vi "Object_Track_Webcam_RIO.vi"() -> ()   [LabVIEW 2017]
doc: "This example demonstrates the Traditional MeanShift algorithm to track an object in the image."
uses:
  <vilib>/NI_Real-Time Target Support.lvlib
panel:
  out "CPU Load":dbl(graph)
  in  "AVI File Path":path=path "/home/lvuser/Traffic.avi"
  in  "Stop":bool
  in  "Delay (s.)":dbl(slide)=0.2040816326530612 scale=0.0..2.0
  out "Image":T1(plugin-control)
  # "Overview: Demonstrate the Traditional MeanShift algorithm to track an object in the image.\nRequirements: LabVIEW Full Development System and Vision Development Module.\nInstructions: Run the VI."
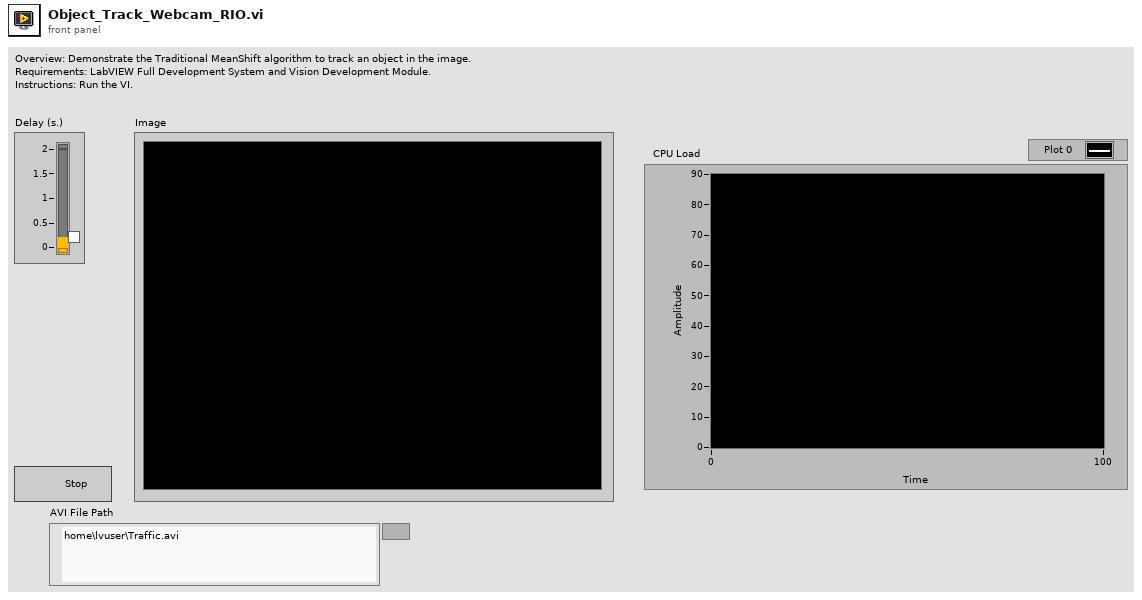
[diagram p1: front panel]
types:
  T1 = typedef "IMAQ Image.ctl" = refnum<image>
  T2 = cluster{"Number of Histogram Bins":i32, "Blending Parameter (%)":dbl, "Maximum Iterations":i32}
  T3 = typedef "IMAQ Object Tracking Session.ctl" = refnum<k20>
  T4 = typedef "IMAQ AVI2 Refnum.ctl" = refnum<k20>
  T5 = typedef "Image Type" = u32
  T6 = typedef "IMAQ Rectangle" = cluster{"Left":i32, "Top":i32, "Right":i32, "Bottom":i32, "Rotation":dbl}
  T7 = typedef "ROI Descriptor" = cluster{"Global Rectangle":i32[], "Contours":cluster{"ID":enum32{"External", "Internal"}, "Type":u32, "Coordinates":i32[]}[]}
  T8 = cluster{"Label":string, "Score":i32, "Angle":dbl, "Location":cluster{"X":dbl, "Y":dbl}, "Bounding Box":cluster{"X":dbl, "Y":dbl}[], "Object Found?":bool}[]
  T9 = cluster{"Label":string, "Score":i32, "Angle":dbl, "Location":cluster{"X":dbl, "Y":dbl}, "Bounding Box":cluster{"X":dbl, "Y":dbl}[], "Object Found?":bool}
  T10 = typedef "NI_Real-Time Target Support.lvlib/RT CPU Load.ctl" = cluster{"Total (%)":dbl, "Time Critical (%)":dbl, "Timed Structures (%)":dbl, "High (%)":dbl, "Above Normal (%)":dbl, "Normal (%)":dbl, "Background (%)":dbl, "Idle (%)":dbl, "ISR (%)":dbl}
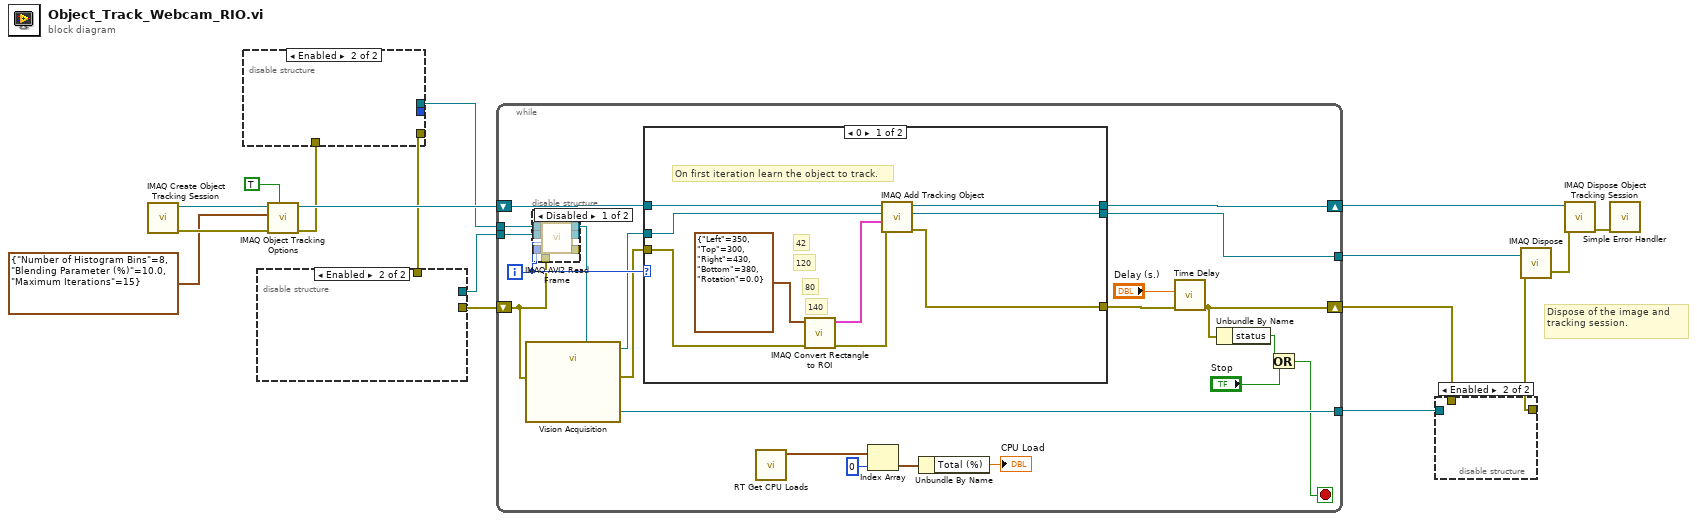
[diagram p0: block diagram]
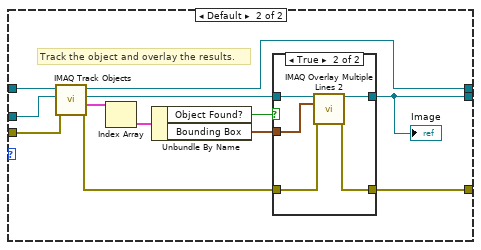
[diagram p3: hidden frame]
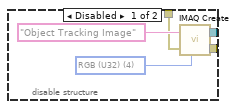
[diagram p5: hidden frame]
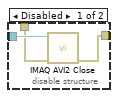
[diagram p6: hidden frame]
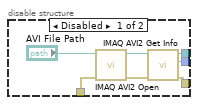
[diagram p7: hidden frame]
diagram:
  # "Dispose of the image and tracking session."
  n1 = call "IMAQ Create Object Tracking Session"() -> ("error out"=w10:errorcluster, "Object Tracking Session"=w13:T3)  [unwired: 1 in, 9 out]
  n2 = call-poly "IMAQ Object Tracking Options"("Get/Set (Get)"=TRUE, "error in (no error)"=w10, "Mean Shift Options in"=T2 {"Number of Histogram Bins"=8, "Blending Parameter (%)"=10.0, "Maximum Iterations"=15}, "Object Tracking Session In"=w13) -> ("error out"=w9:errorcluster, "Object Tracking Session Out"=w12:T3)  [unwired: 5 in, 1 out]
  n3 = disable-structure shown="Enabled" {
    disable-tunnel: w9 -> [w24 _]
    disable-tunnel: [w21 _] -> _
    disable-tunnel: [w20 _] -> w8
    disable-tunnel: [w19 _] -> w7
    frame Disabled {
      n4 = call "IMAQ AVI2 Open"("error in (no error)"=w24, "AVI File Path"="AVI File Path") -> ("error out"=w22:errorcluster, "AVI Refnum"=w23:T4)  [unwired: 8 in]
      n5 = call "IMAQ AVI2 Get Info"("error in (no error)"=w22, "AVI Refnum"=w23) -> ("error out"=w20:errorcluster, "Number of Frames"=w21:u32, "AVI Refnum (duplicate)"=w19:T4)  [unwired: 5 in, 2 out]
    }
    frame Enabled {
    }
  }
  n6 = disable-structure shown="Enabled" {
    disable-tunnel: w8 -> [w28 _]
    disable-tunnel: [w26 _] -> w6
    disable-tunnel: [w25 _] -> w5
    frame Disabled {
      w27 = T5 4 items=["Grayscale (U8)", "Grayscale (I16)", "Grayscale (SGL)", "Complex (CSG)", "RGB (U32)", "HSL (U32)", "RGB (U64)", "Grayscale (U16)"] ("Image Type")
      n7 = call "IMAQ Create"("Image Name"="Object Tracking Image", "Image Type"=w27, "error in (no error)"=w28) -> ("New Image"=w26:T1, "error out"=w25:errorcluster)  [unwired: 2 in]
    }
    frame Enabled {
    }
  }
  n8 = while {
    tunnel: [w48] -> w17
    shift-right: [w46] -> w16
    shift-left: w12 -> [w47]
    tunnel: w7 -> [w44]
    tunnel: w6 -> [w43]
    shift-right: [w32] -> w3
    shift-left: w5 -> [w35]
    tunnel: [w40] -> w4
    i -> [w42]
    stop <- w31 stop-if-true
    n9 = call "Vision Acquisition"("error in"=w35) -> ("Image Out"=w34:T1, "error out"=w33:errorcluster)  [unwired: 24 in, 1 out]
    n10 = disable-structure shown="Disabled" {
      disable-tunnel: w44 -> [w56 _]
      disable-tunnel: w43 -> [w55 _]
      disable-tunnel: [w54 _] -> _
      disable-tunnel: [w53 _] -> _
      disable-tunnel: w42 -> [w52 _]
      disable-tunnel: w35 -> [w51 _]
      disable-tunnel: [w50 _] -> w40
      frame Disabled {
        n11 = call "IMAQ AVI2 Read Frame"("error in (no error)"=w51, "Frame Number"=w52, "Image"=w55, "AVI Refnum"=w56) -> ("error out"=w53:errorcluster, "Image Out"=w54:T1, "AVI Refnum (duplicate)"=w50:T4)  [unwired: 5 in]
      }
      frame Enabled {
      }
    }
    n12 = case shown="0" w42 {
      tunnel: [w62 w77] -> w46
      tunnel: [w64 w74] -> w48
      tunnel: [w63 w70] -> w30
      tunnel: w47 -> [w65 w72]
      tunnel: w34 -> [w61 w68]
      tunnel: w33 -> [w60 w67]
      frame 0 {
        # "140"
        # "80"
        # "42"
        # "120"
        # "On first iteration learn the object to track."
        n13 = call "IMAQ Convert Rectangle to ROI"("error in (no error)"=w60, "Rectangle"=T6 {"Left"=350, "Top"=300, "Right"=430, "Bottom"=380, "Rotation"=0.0}) -> ("error out"=w59:errorcluster, "ROI Descriptor"=w58:T7)  [unwired: 7 in]
        n14 = call "IMAQ Add Tracking Object"("error in (no error)"=w59, "ROI Descriptor"=w58, "Image"=w61, "Object Tracking Session In"=w65) -> ("error out"=w63:errorcluster, "Image (duplicate)"=w64:T1, "Object Tracking Session Out"=w62:T3)  [unwired: 1 in, 4 out]
      }
      frame Default {
        # "Track the object and overlay the results."
        n15 = call "IMAQ Track Objects"("error in (no error)"=w67, "Image"=w68, "Object Tracking Session In"=w72) -> ("error out"=w71:errorcluster, "Objects (pixel)"=w76:T8, "Image (duplicate)"=w75:T1, "Object Tracking Session Out"=w77:T3)  [unwired: 1 in, 4 out]
        n16 = Index Array(array=w76) -> (element=w69:T9)  [unwired: 1 in]
        n17 = Unbundle By Name(w69) -> ("Object Found?"=w66:bool, "Bounding Box"=w73:cluster{"X":dbl, "Y":dbl}[])
        n18 = case shown="True" w66 {
          tunnel: w75 -> [w78 w84]
          tunnel: [w78 w83] -> w74
          tunnel: w73 -> [_ w82]
          tunnel: w71 -> [w79 w81]
          tunnel: [w79 w80] -> w70
          frame False {
          }
          frame True {
            n19 = call "IMAQ Overlay Multiple Lines 2"("Image"=w84, "Line End Points"=w82, "error in (no error)"=w81) -> ("Image Out"=w83:T1, "error out"=w80:errorcluster)  [unwired: 5 in, 6 out]
          }
        }
        "Image" <- w74
      }
    }
    n20 = call <vilib>:"RT Get CPU Loads.vi"() -> ("CPU loads"=w37:T10[])  [unwired: 10 in, 1 out]
    n21 = Index Array(array=w37, index=0) -> (element=w38:T10)
    n22 = Unbundle By Name(w38) -> ("Total (%)"=→"CPU Load":dbl)
    n23 = call "Time Delay"("error in (no error)"=w30, "Delay Time (s)"="Delay (s.)") -> ("error out"=w32:errorcluster)  [unwired: 9 in]
    n24 = Unbundle By Name(w32) -> ("status"=w49:bool)
    n25 = Or(x=w49, y="Stop") -> (x .or. y?=w31:bool)
  }
  n26 = disable-structure shown="Enabled" {
    disable-tunnel: w4 -> [w87 _]
    disable-tunnel: w3 -> [w86 _]
    disable-tunnel: [w85 _] -> w2
    frame Disabled {
      n27 = call "IMAQ AVI2 Close"("error in (no error)"=w86, "AVI Refnum"=w87) -> ("error out"=w85:errorcluster)  [unwired: 9 in]
    }
    frame Enabled {
    }
  }
  n28 = call "IMAQ Dispose"("Image"=w17, "error in (no error)"=w2) -> ("error out"=w15:errorcluster)  [unwired: 1 in, 3 out]
  n29 = call "IMAQ Dispose Object Tracking Session"("error in (no error)"=w15, "Object Tracking Session"=w16) -> ("error out"=w14:errorcluster)  [unwired: 9 out]
  n30 = call <vilib>:"Simple Error Handler.vi"("error in (no error)"=w14) -> ()  [unwired: 1 in, 8 out]
